vi "MenuHandler.vi"(5 "tree control":refnum<vi>, 7 "message queue out":T1, 8 "error in":errorcluster, 9 "parameters":variant, 10 "menu string":string, 11 "module editor node in":refnum<class "module editor node.lvclass">) -> (0 "error out":errorcluster, 2 "Unhandled":bool, 3 "module editor node out":refnum<class "module editor node.lvclass">)   [LabVIEW 2013, in "PL Framework Configuration Tool.lvlib" / "module editor node.lvclass"]
uses:
  module editor node.lvclass
  <vilib>/NI/AMC/Message Queue.ctl
  <vilib>/NI/AMC/Message.ctl
  <vilib>/NI/Tools/Keyed Array/KeyedArray.ctl
  TBM Configuration Node/TBM Configuration Node.lvclass
  <vilib>/NI/AMC/Create Single Message.vi
  <vilib>/NI/AMC/Update Message Routing Info.vi
  <vilib>/NI/AMC/Send Message.vi
  <vilib>/NI/AMC/AMC.lvlib
  <vilib>/NI/Tools/Keyed Array/Tools_KeyedArray.lvlib
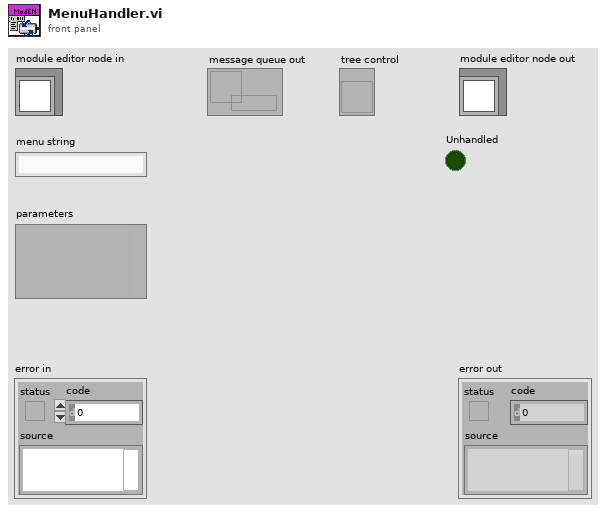
[diagram p1: front panel]
types:
  T1 = typedef "AMC.lvlib/Message Queue.ctl" = refnum<queue>
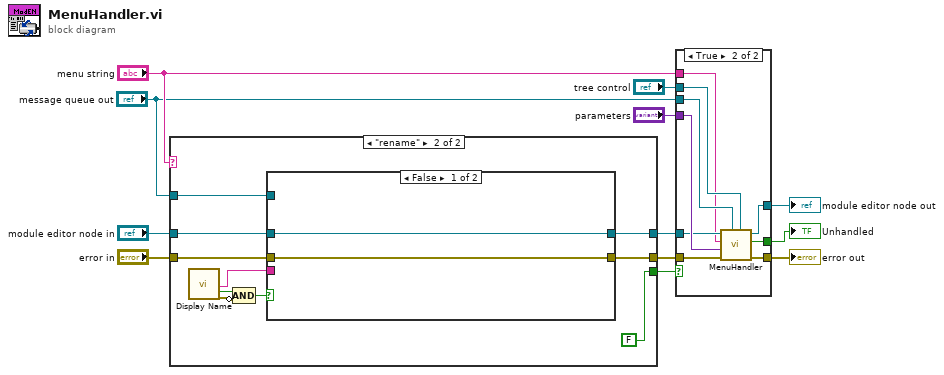
[diagram p0: block diagram]
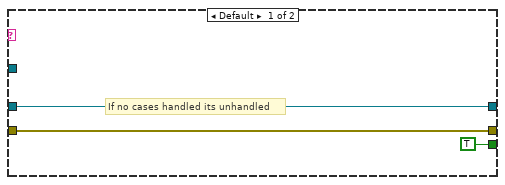
[diagram p3: hidden frame]
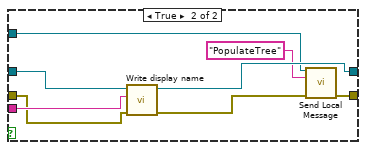
[diagram p4: hidden frame]
diagram:
  n1 = case shown="\"rename\"" "menu string" {
    tunnel: [TRUE ("Unhandled") FALSE ("Unhandled")] -> w3
    tunnel: "module editor node in" -> [w14 w22]
    tunnel: [w14 w21] -> w6
    tunnel: [w13 w23] -> w5
    tunnel: "error in" -> [w13 w24]
    tunnel: "message queue out" -> [_ w16]
    frame Default {
      # "If no cases handled its unhandled"
    }
    frame "rename" {
      n2 = call "Display Name"() -> ("Display Name"=w17:string, "OK"=w20:bool, "error out"=w19:errorcluster)  [unwired: 17 in]
      n3 = Compound Arithmetic op=AND(w20, invert w19) -> (w18:bool)
      n4 = case shown="False" w18 {
        tunnel: w24 -> [w26 w28]
        tunnel: [w26 w31] -> w23
        tunnel: w22 -> [w27 w35]
        tunnel: [w27 w34] -> w21
        tunnel: w17 -> [_ w29]
        tunnel: w16 -> [_ w30]
        frame False {
        }
        frame True {
          n5 = call "Write display name.vi"("error in"=w28, "display name"=w29, "module editor node in"=w35) -> ("error out"=w32:errorcluster, "module editor node out"=w34:refnum<class "module editor node.lvclass">)  [unwired: 7 in]
          n6 = call <vilib>:"Send Local Message.vi"("message queue in"=w30, "message name"="PopulateTree", "error in"=w32) -> ("error out"=w31:errorcluster)  [unwired: 10 in, 2 out]
        }
      }
    }
  }
  n7 = case shown="True" w3 {
    selector: w3 -> [w38 _]
    tunnel: [w36 w47] -> w12
    tunnel: [w38 w46] -> w11
    tunnel: [w37 w45] -> w10
    tunnel: "tree control" -> [_ w44]
    tunnel: "message queue out" -> [_ w43]
    tunnel: "parameters" -> [_ w42]
    tunnel: w6 -> [w37 w41]
    tunnel: w5 -> [w36 w40]
    tunnel: "menu string" -> [_ w39]
    frame False {
    }
    frame True {
      n8 = call-parent "MenuHandler.vi"("tree control"=w44, "message queue out"=w43, "error in (no error)"=w40, "parameters"=w42, "menu string"=w39, "NISE_CEF_Node in"=w41) -> ("error out"=w47:errorcluster, "Unhandled"=w46:bool, "NISE_CEF_Node out"=w45:refnum<class "module editor node.lvclass">)  [unwired: 3 in]
    }
  }
  "error out" <- w12
  "module editor node out" <- w10
  "Unhandled" <- w11
